vi "client_player.vi"() -> ()   [LabVIEW 2020]
panel:
  in  "LEVEL":i32(slide)=3000 scale=5.0..1.0
  out "Int32":i32
  out "Tank":i32(slide)
  in  "Boolean":bool
  in  "Boolean 3":bool
  in  "Boolean 4":bool
  in  "Boolean 5":bool
  in  "Boolean 6":bool
  in  "Boolean 7":bool
  in  "Boolean 8":bool
  in  "Boolean 9":bool
  in  "Boolean 2":bool
  in  "stop":bool
  out "XO array":string[][](array[string])
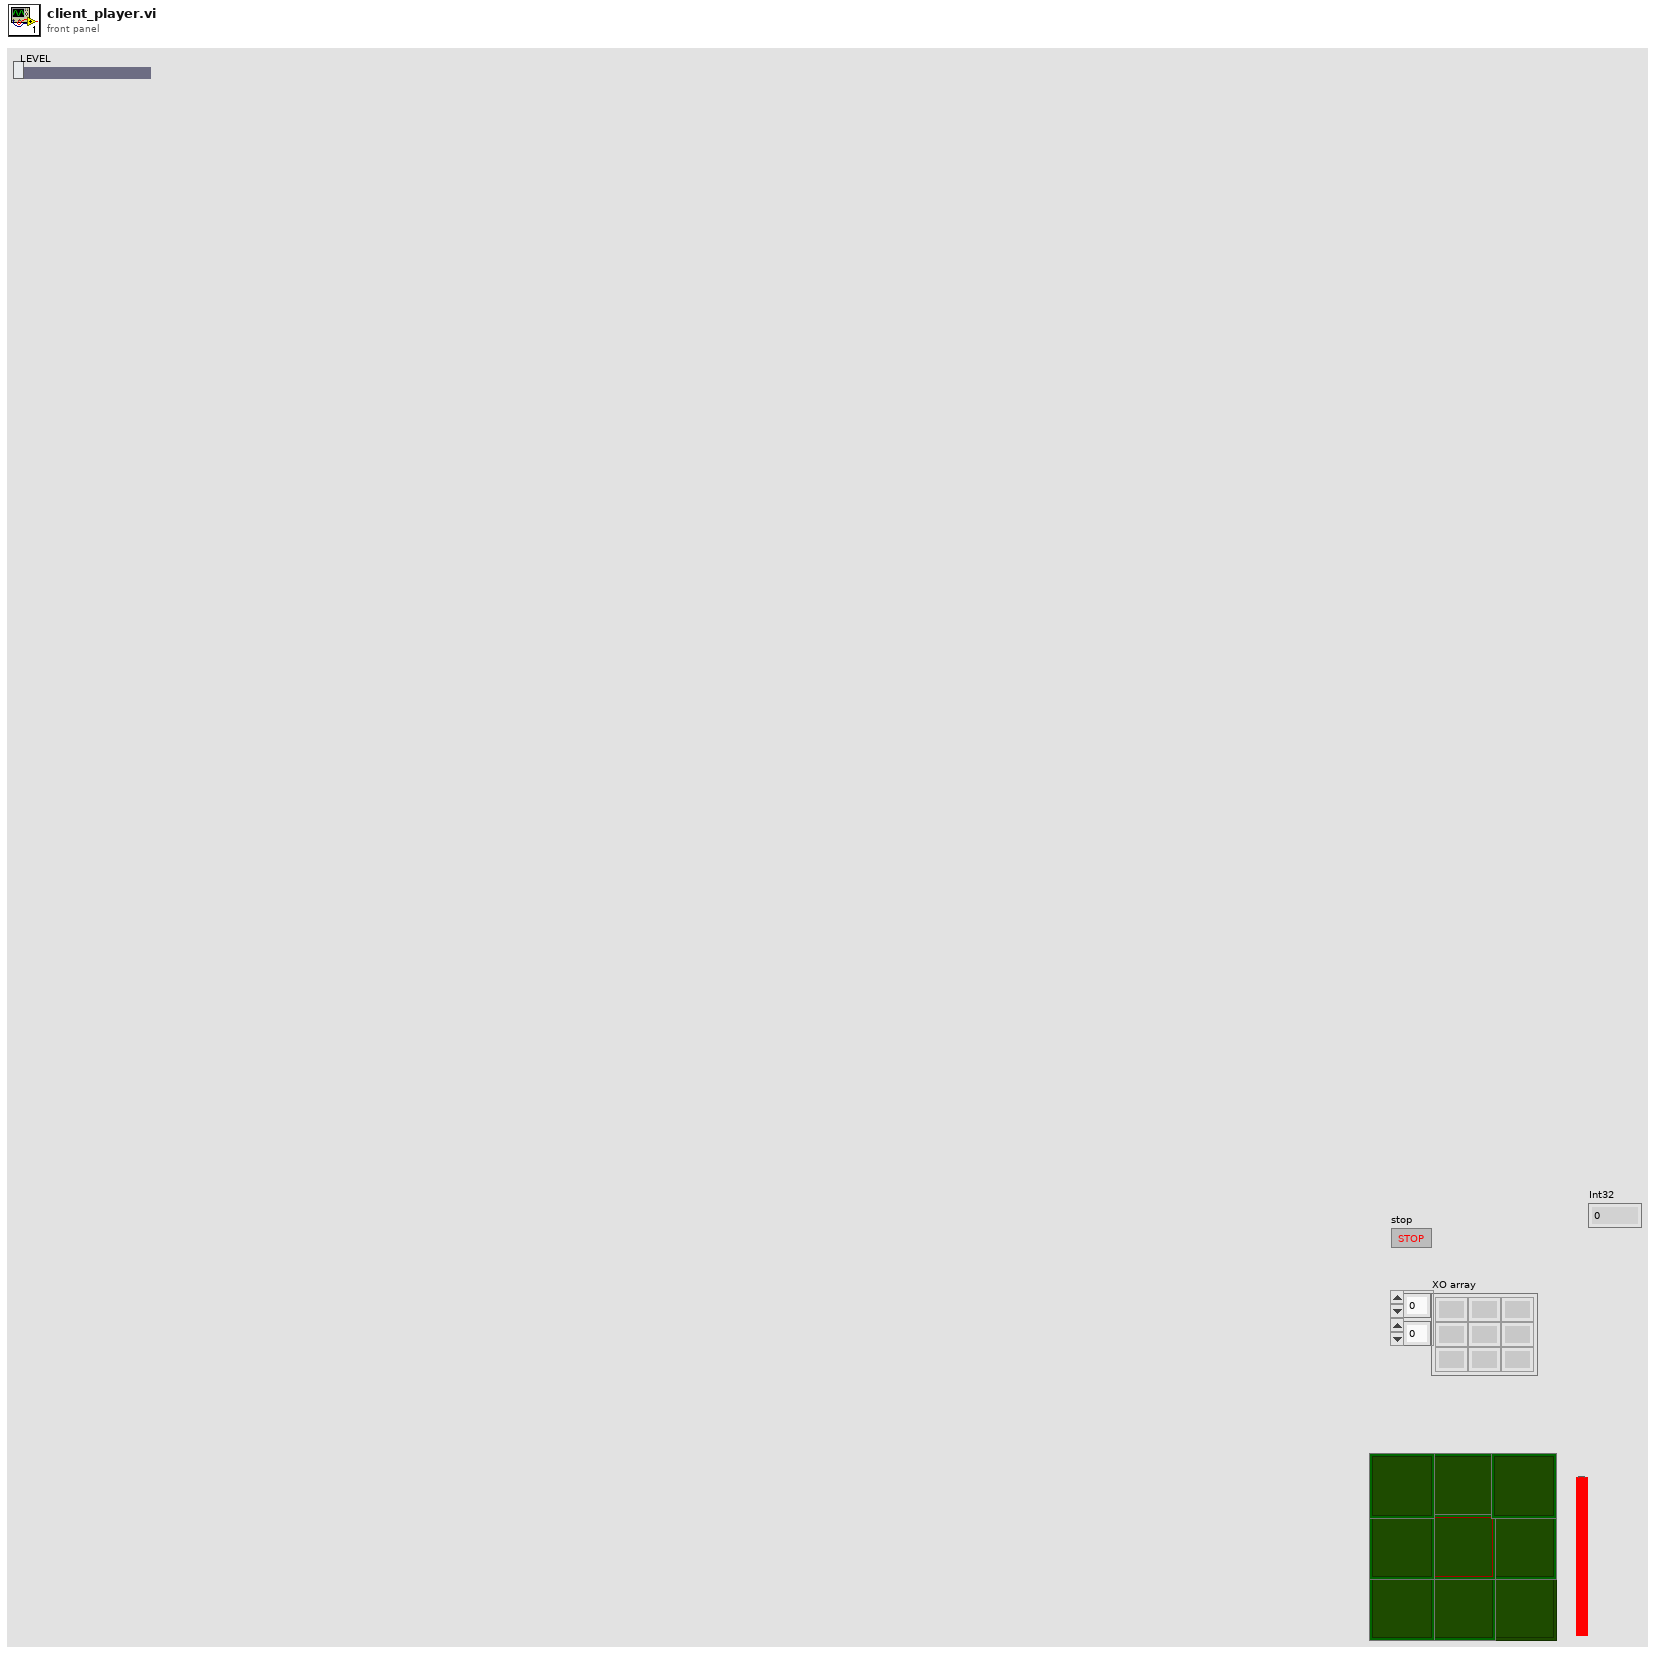
[diagram p1: front panel]
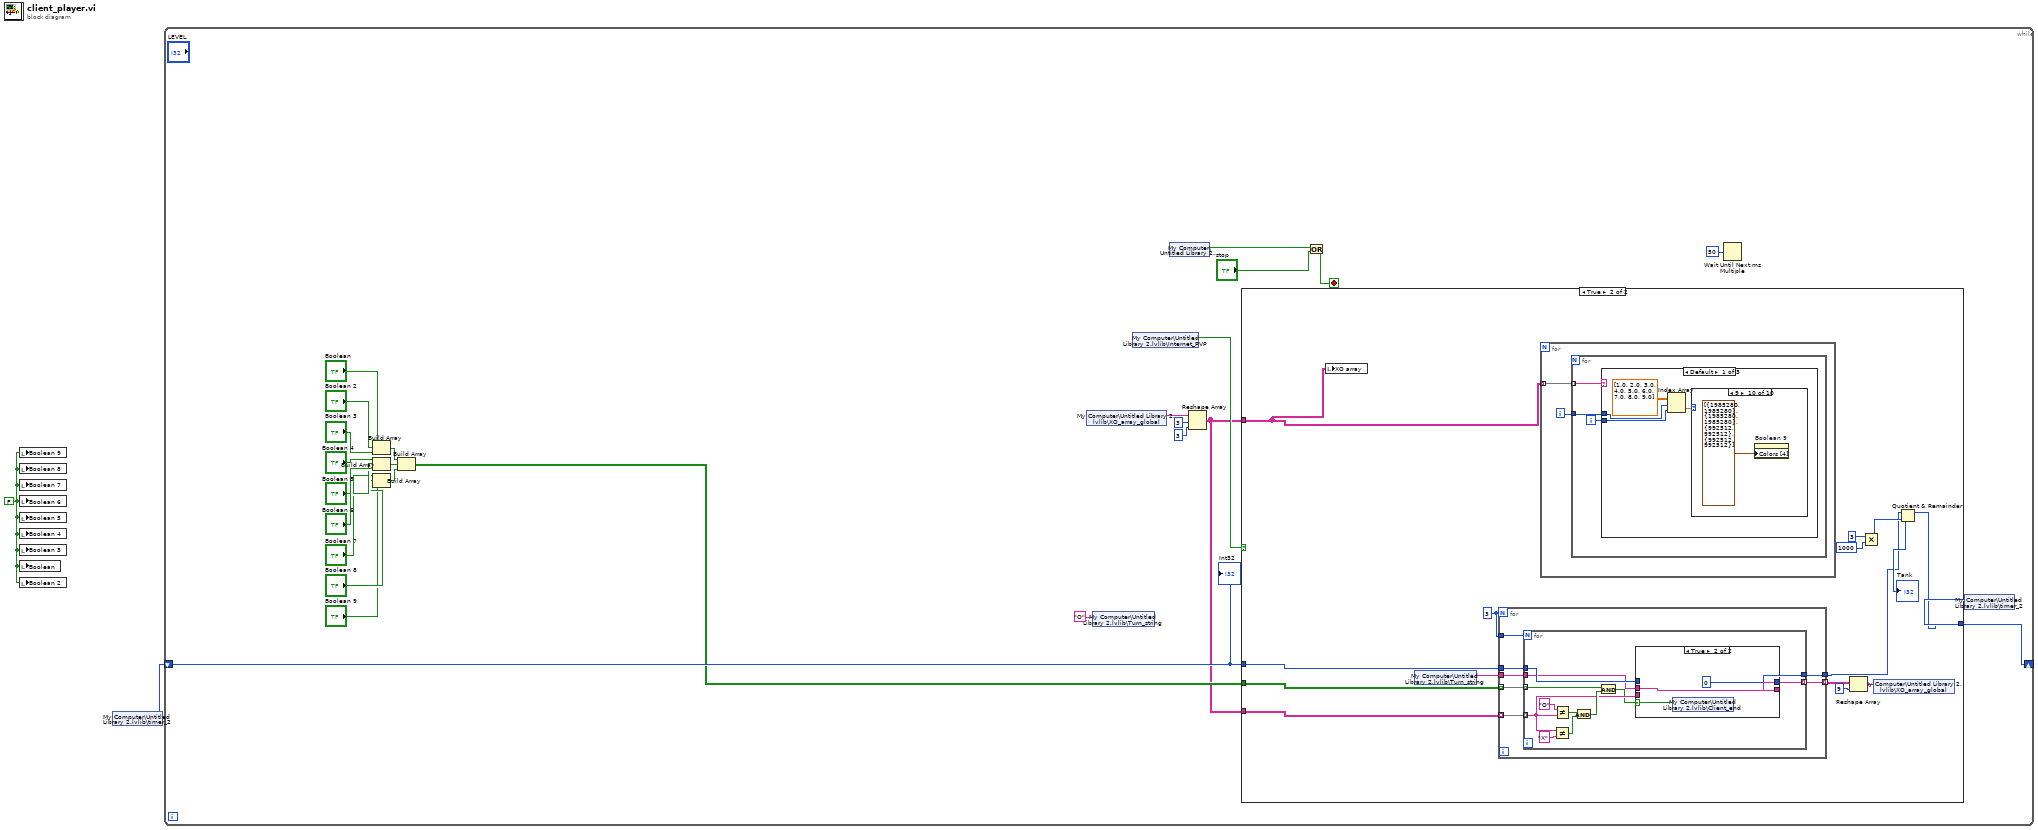
[diagram p0: block diagram]
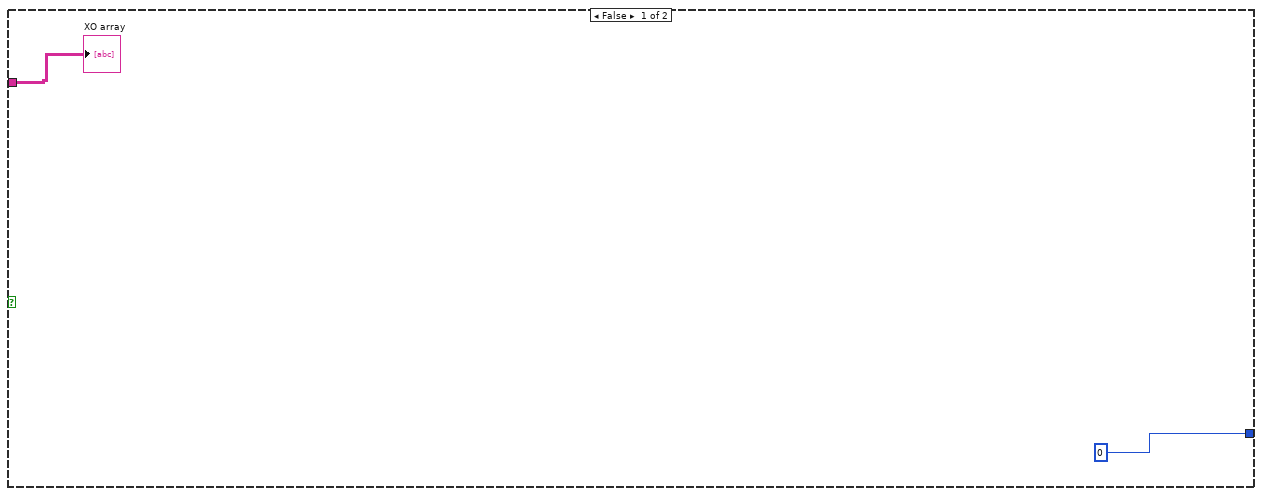
[diagram p2: hidden frame]
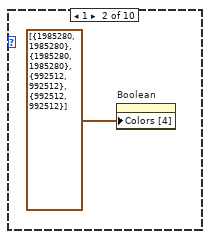
[diagram p4: hidden frame]
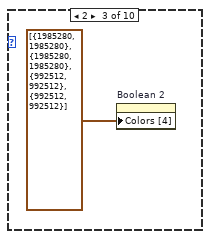
[diagram p5: hidden frame]
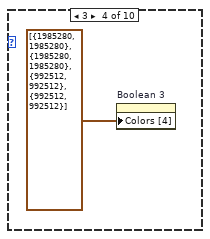
[diagram p6: hidden frame]
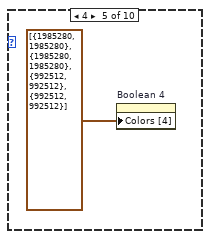
[diagram p7: hidden frame]
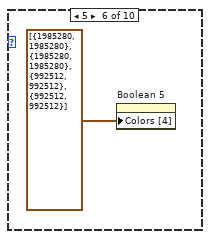
[diagram p8: hidden frame]
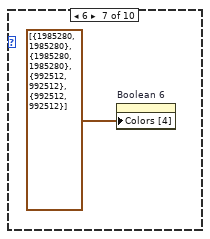
[diagram p9: hidden frame]
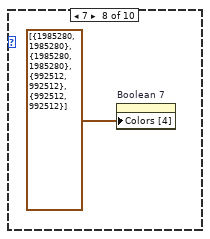
[diagram p10: hidden frame]
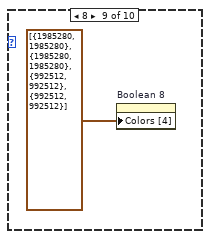
[diagram p11: hidden frame]
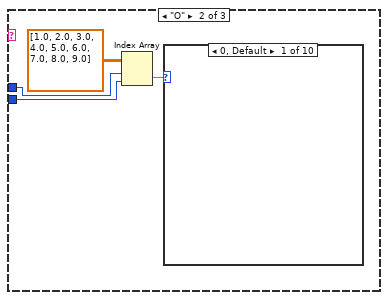
[diagram p12: hidden frame]
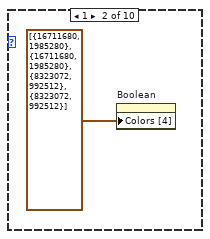
[diagram p13: hidden frame]
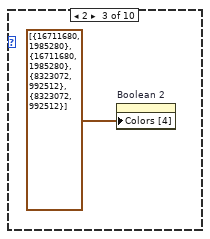
[diagram p14: hidden frame]
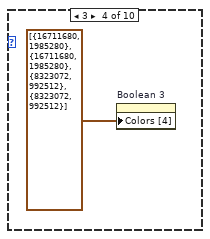
[diagram p15: hidden frame]
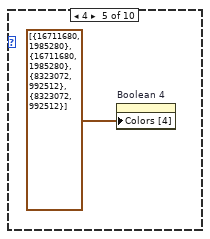
[diagram p16: hidden frame]
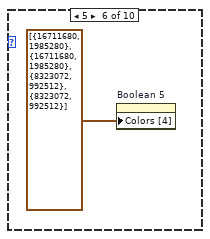
[diagram p17: hidden frame]
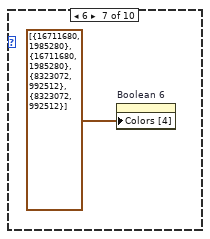
[diagram p18: hidden frame]
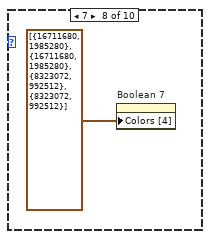
[diagram p19: hidden frame]
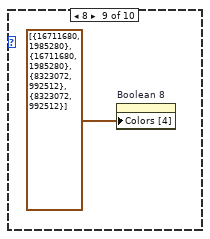
[diagram p20: hidden frame]
diagram:
  w1 = FALSE
  n1 = local write "Boolean 9"(w1) -> ()
  n2 = local write "Boolean 8"(w1) -> ()
  n3 = local write "Boolean 7"(w1) -> ()
  n4 = local write "Boolean 6"(w1) -> ()
  n5 = local write "Boolean 5"(w1) -> ()
  n6 = local write "Boolean 4"(w1) -> ()
  n7 = local write "Boolean 3"(w1) -> ()
  n8 = local write "Boolean"(w1) -> ()
  n9 = local write "Boolean 2"(w1) -> ()
  n10 = shared-variable "My Computer\\Untitled Library 2.lvlib\\timer_2"() -> (w2:i32)  [unwired: 1 in, 1 out]
  n11 = while {
    shift-right: [w8] -> _
    shift-left: w2 -> [w24]
    stop <- w26 stop-if-true
    n12 = Build Array("Boolean", "Boolean 2", "Boolean 3") -> (w21:bool[])
    n13 = Build Array("Boolean 4", "Boolean 5", "Boolean 6") -> (w22:bool[])
    n14 = Build Array("Boolean 7", "Boolean 8", "Boolean 9") -> (w23:bool[])
    n15 = Build Array(w21, w22, w23) -> (w12:bool[][])
    n16 = shared-variable "My Computer\\Untitled Library 2.lvlib\\XO_array_global"() -> (w7:string[])  [unwired: 1 in, 1 out]
    n17 = shared-variable "My Computer\\Untitled Library 2.lvlib\\Turn_string"("O" ("x")) -> ()  [unwired: 1 in, 1 out]
    n18 = shared-variable "My Computer\\Untitled Library 2.lvlib\\Internet_PVP"() -> (w10:bool)  [unwired: 1 in, 1 out]
    n19 = shared-variable "My Computer\\Untitled Library 2.lvlib\\stop"() -> (w27:bool)  [unwired: 1 in, 1 out]
    n20 = Reshape Array(w7, 3 ("dimension size"), 3 ("dimension size")) -> (w4:string[][])
    n21 = case shown="True" w10 {
      tunnel: w24 -> [_ w43]
      tunnel: w12 -> [_ w42]
      tunnel: [0 ("Int32") w41] -> w8
      tunnel: w4 -> [_ w40]
      tunnel: w4 -> [w28 w30]
      frame False {
        "XO array" <- w28
      }
      frame True {
        w39 = 3
        n22 = local write "XO array"(w30) -> ()
        n23 = shared-variable "My Computer\\Untitled Library 2.lvlib\\Turn_string"() -> (w38:string)  [unwired: 1 in, 1 out]
        n24 = for {
          N: w39 -> [_]
          tunnel: w39 -> [w94]
          tunnel: w42 -> [w93] mode=indexing
          tunnel: w40 -> [w92] mode=indexing
          tunnel: [w91] -> w37 mode=indexing
          tunnel: w43 -> [w90]
          tunnel: [w89] -> w33
          tunnel: w38 -> [w88]
          n25 = for {
            N: w94 -> [_]
            tunnel: w93 -> [w102] mode=indexing
            tunnel: w92 -> [w100] mode=indexing
            tunnel: [w99] -> w91 mode=indexing
            tunnel: w90 -> [w97]
            tunnel: [w96] -> w89
            tunnel: w88 -> [w95]
            n26 = Not Equal?(x=w100, y="X") -> (x != y?=w103:bool)
            n27 = Not Equal?(x="O", y=w100) -> (x != y?=w104:bool)
            n28 = And(x=w104, y=w103) -> (x .and. y?=w101:bool)
            n29 = And(x=w102, y=w101) -> (x .and. y?=w98:bool)
            n30 = case shown="True" w98 {
              selector: w98 -> [_ w110]
              tunnel: w100 -> [w109 _]
              tunnel: [w109 w111] -> w99
              tunnel: w97 -> [w108 _]
              tunnel: [w107 0] -> w96
              tunnel: w95 -> [_ w111]
              frame False {
                n31 = Increment(x=w108) -> (x+1=w107:i32)
              }
              frame True {
                n32 = shared-variable "My Computer\\Untitled Library 2.lvlib\\Client_end"(w110) -> ()  [unwired: 1 in, 1 out]
              }
            }
          }
        }
        n33 = for {
          tunnel: w30 -> [w44] mode=indexing
          i -> [w45]
          n34 = for {
            tunnel: w45 -> [w48]
            tunnel: w44 -> [w46] mode=indexing
            i -> [w47]
            n35 = case shown="Default" w46 {
              tunnel: w48 -> [w52 w63 w76]
              tunnel: w47 -> [w51 w62 w77]
              frame Default {
                n36 = Index Array(array=dbl[][] [[1.0, 2.0, 3.0], [4.0, 5.0, 6.0], [7.0, 8.0, 9.0]] ("Array"), index (row)=w52, index (col)=w51) -> (element=w49:dbl)
                n37 = case shown="9" w49 {
                  frame 0, Default {
                  }
                  frame 1 {
                    n38 = property on="Boolean" class="Bool (strict)"("Colors [4]"=cluster{u32, u32}[] [{1985280, 1985280}, {1985280, 1985280}, {992512, 992512}, {992512, 992512}]) -> ()  [unwired: 2 in, 2 out]
                  }
                  frame 2 {
                    n39 = property on="Boolean 2" class="Bool (strict)"("Colors [4]"=cluster{u32, u32}[] [{1985280, 1985280}, {1985280, 1985280}, {992512, 992512}, {992512, 992512}]) -> ()  [unwired: 2 in, 2 out]
                  }
                  frame 3 {
                    n40 = property on="Boolean 3" class="Bool (strict)"("Colors [4]"=cluster{u32, u32}[] [{1985280, 1985280}, {1985280, 1985280}, {992512, 992512}, {992512, 992512}]) -> ()  [unwired: 2 in, 2 out]
                  }
                  frame 4 {
                    n41 = property on="Boolean 4" class="Bool (strict)"("Colors [4]"=cluster{u32, u32}[] [{1985280, 1985280}, {1985280, 1985280}, {992512, 992512}, {992512, 992512}]) -> ()  [unwired: 2 in, 2 out]
                  }
                  frame 5 {
                    n42 = property on="Boolean 5" class="Bool (strict)"("Colors [4]"=cluster{u32, u32}[] [{1985280, 1985280}, {1985280, 1985280}, {992512, 992512}, {992512, 992512}]) -> ()  [unwired: 2 in, 2 out]
                  }
                  frame 6 {
                    n43 = property on="Boolean 6" class="Bool (strict)"("Colors [4]"=cluster{u32, u32}[] [{1985280, 1985280}, {1985280, 1985280}, {992512, 992512}, {992512, 992512}]) -> ()  [unwired: 2 in, 2 out]
                  }
                  frame 7 {
                    n44 = property on="Boolean 7" class="Bool (strict)"("Colors [4]"=cluster{u32, u32}[] [{1985280, 1985280}, {1985280, 1985280}, {992512, 992512}, {992512, 992512}]) -> ()  [unwired: 2 in, 2 out]
                  }
                  frame 8 {
                    n45 = property on="Boolean 8" class="Bool (strict)"("Colors [4]"=cluster{u32, u32}[] [{1985280, 1985280}, {1985280, 1985280}, {992512, 992512}, {992512, 992512}]) -> ()  [unwired: 2 in, 2 out]
                  }
                  frame 9 {
                    n46 = property on="Boolean 9" class="Bool (strict)"("Colors [4]"=cluster{u32, u32}[] [{1985280, 1985280}, {1985280, 1985280}, {992512, 992512}, {992512, 992512}]) -> ()  [unwired: 2 in, 2 out]
                  }
                }
              }
              frame "O" {
                n47 = Index Array(array=dbl[][] [[1.0, 2.0, 3.0], [4.0, 5.0, 6.0], [7.0, 8.0, 9.0]] ("Array"), index (row)=w63, index (col)=w62) -> (element=w64:dbl)
                n48 = case shown="0, Default" w64 {
                  frame 0, Default {
                  }
                  frame 1 {
                    n49 = property on="Boolean" class="Bool (strict)"("Colors [4]"=cluster{u32, u32}[] [{16711680, 1985280}, {16711680, 1985280}, {8323072, 992512}, {8323072, 992512}]) -> ()  [unwired: 2 in, 2 out]
                  }
                  frame 2 {
                    n50 = property on="Boolean 2" class="Bool (strict)"("Colors [4]"=cluster{u32, u32}[] [{16711680, 1985280}, {16711680, 1985280}, {8323072, 992512}, {8323072, 992512}]) -> ()  [unwired: 2 in, 2 out]
                  }
                  frame 3 {
                    n51 = property on="Boolean 3" class="Bool (strict)"("Colors [4]"=cluster{u32, u32}[] [{16711680, 1985280}, {16711680, 1985280}, {8323072, 992512}, {8323072, 992512}]) -> ()  [unwired: 2 in, 2 out]
                  }
                  frame 4 {
                    n52 = property on="Boolean 4" class="Bool (strict)"("Colors [4]"=cluster{u32, u32}[] [{16711680, 1985280}, {16711680, 1985280}, {8323072, 992512}, {8323072, 992512}]) -> ()  [unwired: 2 in, 2 out]
                  }
                  frame 5 {
                    n53 = property on="Boolean 5" class="Bool (strict)"("Colors [4]"=cluster{u32, u32}[] [{16711680, 1985280}, {16711680, 1985280}, {8323072, 992512}, {8323072, 992512}]) -> ()  [unwired: 2 in, 2 out]
                  }
                  frame 6 {
                    n54 = property on="Boolean 6" class="Bool (strict)"("Colors [4]"=cluster{u32, u32}[] [{16711680, 1985280}, {16711680, 1985280}, {8323072, 992512}, {8323072, 992512}]) -> ()  [unwired: 2 in, 2 out]
                  }
                  frame 7 {
                    n55 = property on="Boolean 7" class="Bool (strict)"("Colors [4]"=cluster{u32, u32}[] [{16711680, 1985280}, {16711680, 1985280}, {8323072, 992512}, {8323072, 992512}]) -> ()  [unwired: 2 in, 2 out]
                  }
                  frame 8 {
                    n56 = property on="Boolean 8" class="Bool (strict)"("Colors [4]"=cluster{u32, u32}[] [{16711680, 1985280}, {16711680, 1985280}, {8323072, 992512}, {8323072, 992512}]) -> ()  [unwired: 2 in, 2 out]
                  }
                  frame 9 {
                    n57 = property on="Boolean 9" class="Bool (strict)"("Colors [4]"=cluster{u32, u32}[] [{16711680, 1985280}, {16711680, 1985280}, {8323072, 992512}, {8323072, 992512}]) -> ()  [unwired: 2 in, 2 out]
                  }
                }
              }
              frame "X" {
                n58 = Index Array(array=dbl[][] [[1.0, 2.0, 3.0], [4.0, 5.0, 6.0], [7.0, 8.0, 9.0]] ("Array"), index (row)=w76, index (col)=w77) -> (element=w78:dbl)
                n59 = case shown="9" w78 {
                  frame 0, Default {
                  }
                  frame 1 {
                    n60 = property on="Boolean" class="Bool (strict)"("Colors [4]"=cluster{u32, u32}[] [{6618880, 6618880}, {6618880, 6618880}, {3309312, 3309312}, {3309312, 3309312}]) -> ()  [unwired: 2 in, 2 out]
                  }
                  frame 2 {
                    n61 = property on="Boolean 2" class="Bool (strict)"("Colors [4]"=cluster{u32, u32}[] [{6618880, 6618880}, {6618880, 6618880}, {3309312, 3309312}, {3309312, 3309312}]) -> ()  [unwired: 2 in, 2 out]
                  }
                  frame 3 {
                    n62 = property on="Boolean 3" class="Bool (strict)"("Colors [4]"=cluster{u32, u32}[] [{6618880, 6618880}, {6618880, 6618880}, {3309312, 3309312}, {3309312, 3309312}]) -> ()  [unwired: 2 in, 2 out]
                  }
                  frame 4 {
                    n63 = property on="Boolean 4" class="Bool (strict)"("Colors [4]"=cluster{u32, u32}[] [{6618880, 6618880}, {6618880, 6618880}, {3309312, 3309312}, {3309312, 3309312}]) -> ()  [unwired: 2 in, 2 out]
                  }
                  frame 5 {
                    n64 = property on="Boolean 5" class="Bool (strict)"("Colors [4]"=cluster{u32, u32}[] [{6618880, 6618880}, {6618880, 6618880}, {3309312, 3309312}, {3309312, 3309312}]) -> ()  [unwired: 2 in, 2 out]
                  }
                  frame 6 {
                    n65 = property on="Boolean 6" class="Bool (strict)"("Colors [4]"=cluster{u32, u32}[] [{6618880, 6618880}, {6618880, 6618880}, {3309312, 3309312}, {3309312, 3309312}]) -> ()  [unwired: 2 in, 2 out]
                  }
                  frame 7 {
                    n66 = property on="Boolean 7" class="Bool (strict)"("Colors [4]"=cluster{u32, u32}[] [{6618880, 6618880}, {6618880, 6618880}, {3309312, 3309312}, {3309312, 3309312}]) -> ()  [unwired: 2 in, 2 out]
                  }
                  frame 8 {
                    n67 = property on="Boolean 8" class="Bool (strict)"("Colors [4]"=cluster{u32, u32}[] [{6618880, 6618880}, {6618880, 6618880}, {3309312, 3309312}, {3309312, 3309312}]) -> ()  [unwired: 2 in, 2 out]
                  }
                  frame 9 {
                    n68 = property on="Boolean 9" class="Bool (strict)"("Colors [4]"=cluster{u32, u32}[] [{6618880, 6618880}, {6618880, 6618880}, {3309312, 3309312}, {3309312, 3309312}]) -> ()  [unwired: 2 in, 2 out]
                  }
                }
              }
            }
          }
        }
        n69 = Reshape Array(w37, 9 ("dimension size")) -> (w36:string[])
        n70 = Multiply(x=3, y=1000) -> (x*y=w34:i32)
        n71 = shared-variable "My Computer\\Untitled Library 2.lvlib\\XO_array_global"(w36) -> ()  [unwired: 1 in, 1 out]
        n72 = Quotient & Remainder(x=w33, y=w34) -> (x-y*floor(x/y)=w41:i32)  [unwired: 1 out]
        "Tank" <- w41
      }
    }
    n73 = Or(x=w27, y="stop") -> (x .or. y?=w26:bool)
    n74 = Wait Until Next ms Multiple(millisecond multiple=u32 50) -> ()  [unwired: 1 out]
    n75 = shared-variable "My Computer\\Untitled Library 2.lvlib\\timer_2"(w8) -> ()  [unwired: 1 in, 1 out]
    "Int32" <- w24
  }
